vi "disable all controls.vi"(6 "DisabledEnum":T1(ring)=enum."Disabled and Grayed Out", 8 "error in":errorcluster, 11 "Cluster in":T2={"This VI Ref"=refnum, "Test VI"=refnum, "Q Ref"=refnum, "UE"=refnum, "Data"=variant, "Timeout"=-1, "Path List[]"=[], "Status"="", "Counter"=0, "Config"={"Source Path"=path "", "Dest Path"=path "", "Log Path"=path "", "Move?"=FALSE, "Log?"=FALSE, "Scanners"=[], "Excude Folders"=[], "Jpg?"=FALSE, "Default path"=path "", "Extended?"=FALSE, "Mode"=enum."Move", "Temp"=FALSE}, "Total"=0, "Config Path"=path "", "exif info"={"Make"="Canon\u0000", "Model"="Canon PowerShot A495\u0000", "Orientation"=0, "Date"=timestamp(0 s since 1904-01-01), "Width"=0, "Height"=0, "Square?"=FALSE, "File Name"="Canon\u0000", "Extension"="Canon\u0000", "Valid?"=FALSE, "Path"=path "", "size"=0, "No Ext?"=FALSE, "prefix?"=FALSE, "String"="", "Name Type"=enum."Event Sufix"}, "app operation"=enum."Start", "Log Ref"=refnum, "Start Time"=0.0, "Pause Time"=0.0, "Argument?"=FALSE, "Argument path"=path "", "Identical"=FALSE, "File.lvclass"=refnum}) -> (0 "error out":errorcluster, 3 "Cluster out":T2={"This VI Ref"=refnum, "Test VI"=refnum, "Q Ref"=refnum, "UE"=refnum, "Data"=variant, "Timeout"=-1, "Path List[]"=[], "Status"="", "Counter"=0, "Config"={"Source Path"=path "", "Dest Path"=path "", "Log Path"=path "", "Move?"=FALSE, "Log?"=FALSE, "Scanners"=[], "Excude Folders"=[], "Jpg?"=FALSE, "Default path"=path "", "Extended?"=FALSE, "Mode"=enum."Move", "Temp"=FALSE}, "Total"=0, "Config Path"=path "", "exif info"={"Make"="Canon\u0000", "Model"="Canon PowerShot A495\u0000", "Orientation"=0, "Date"=timestamp(0 s since 1904-01-01), "Width"=0, "Height"=0, "Square?"=FALSE, "File Name"="Canon\u0000", "Extension"="Canon\u0000", "Valid?"=FALSE, "Path"=path "", "size"=0, "No Ext?"=FALSE, "prefix?"=FALSE, "String"="", "Name Type"=enum."Event Sufix"}, "app operation"=enum."Start", "Log Ref"=refnum, "Start Time"=0.0, "Pause Time"=0.0, "Argument?"=FALSE, "Argument path"=path "", "Identical"=FALSE, "File.lvclass"=refnum})   [LabVIEW 2023, in "User Interface.lvlib"]
uses:
  User Interface.lvlib
  Controls/configuration cluster.ctl
  File Classes/Controls/rename type enum.ctl
  File Classes/File Classes.lvlib
  File Classes/Controls/exif data cluster.ctl
  Controls/app operation state enum.ctl
  File Classes/File/File.lvclass
  Controls/main consumer cluster.ctl
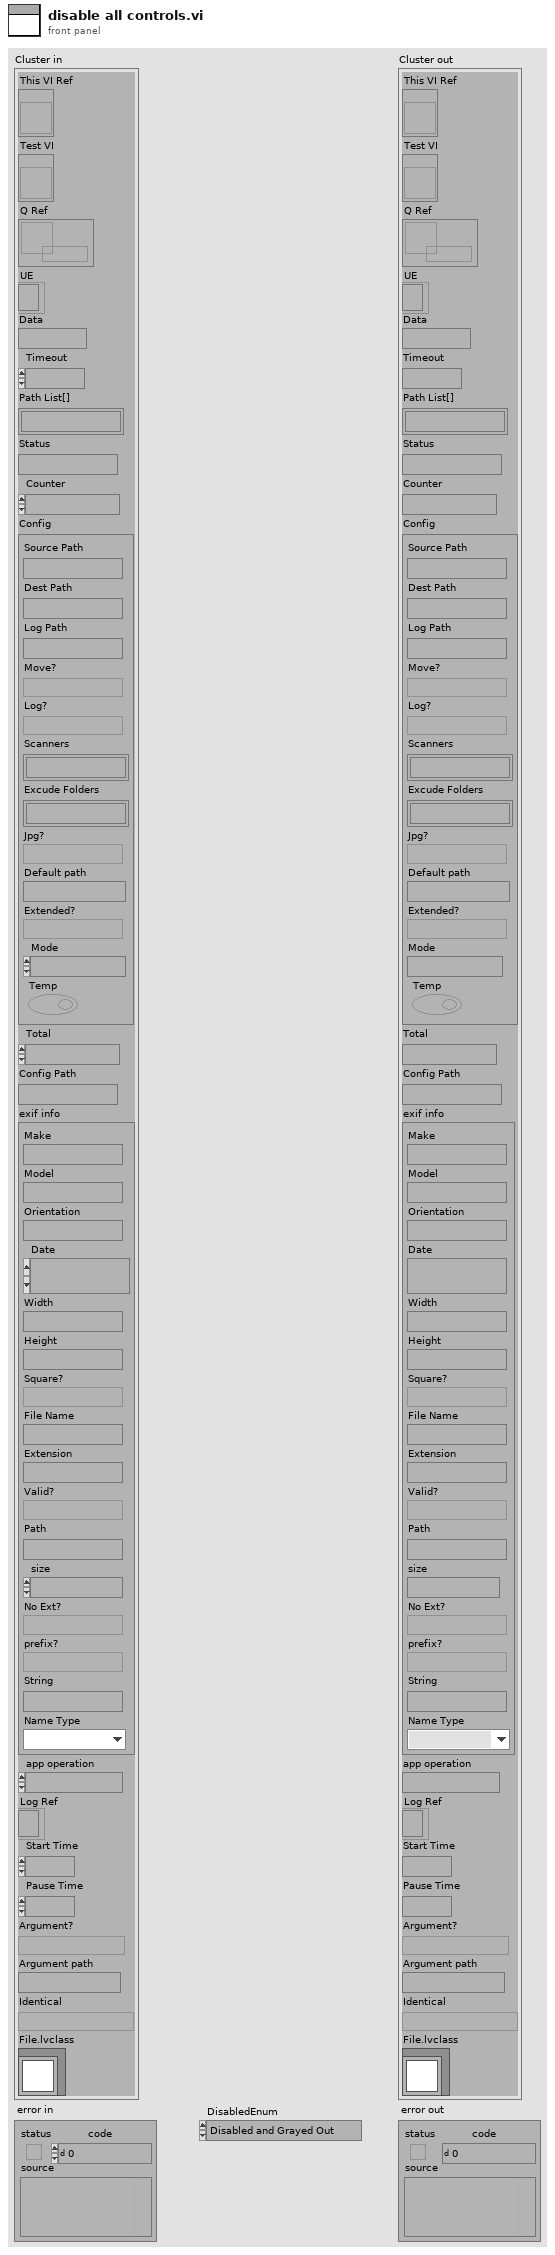
[diagram p1: front panel]
types:
  T1 = enum8{"Enabled", "Disabled", "Disabled and Grayed Out"}
  T2 = typedef "User Interface.lvlib/main consumer cluster.ctl" = cluster{"This VI Ref":refnum<vi>, "Test VI":refnum<vi>, "Q Ref":refnum<queue>, "UE":refnum<event-registration>, "Data":variant, "Timeout":i32, "Path List[]":path[], "Status":string, "Counter":i32, "Config":T3, "Total":i32, "Config Path":path, "exif info":T4, "app operation":T6, "Log Ref":refnum<file>, "Start Time":dbl, "Pause Time":dbl, "Argument?":bool, "Argument path":path, "Identical":bool, "File.lvclass":refnum<class "File.lvclass">}
  T3 = typedef "User Interface.lvlib/configuration cluster.ctl" = cluster{"Source Path":path, "Dest Path":path, "Log Path":path, "Move?":bool, "Log?":bool, "Scanners":string[], "Excude Folders":string[], "Jpg?":bool, "Default path":path, "Extended?":bool, "Mode":enum16{"Copy (Default)", "Move", "Rename"}, "Temp":bool}
  T4 = typedef "File Classes.lvlib/exif data cluster.ctl" = cluster{"Make":string, "Model":string, "Orientation":u16, "Date":timestamp, "Width":u16, "Height":u16, "Square?":bool, "File Name":string, "Extension":string, "Valid?":bool, "Path":path, "size":i64, "No Ext?":bool, "prefix?":bool, "String":string, "Name Type":T5}
  T5 = typedef "File Classes.lvlib/rename type enum.ctl" = enum16{"Date & Time (Default)", "Model Sufix", "Event Sufix", "Model & Event Sufix"}
  T6 = typedef "User Interface.lvlib/app operation state enum.ctl" = enum16{"Start", "Stop", "Pause", "Resume"}
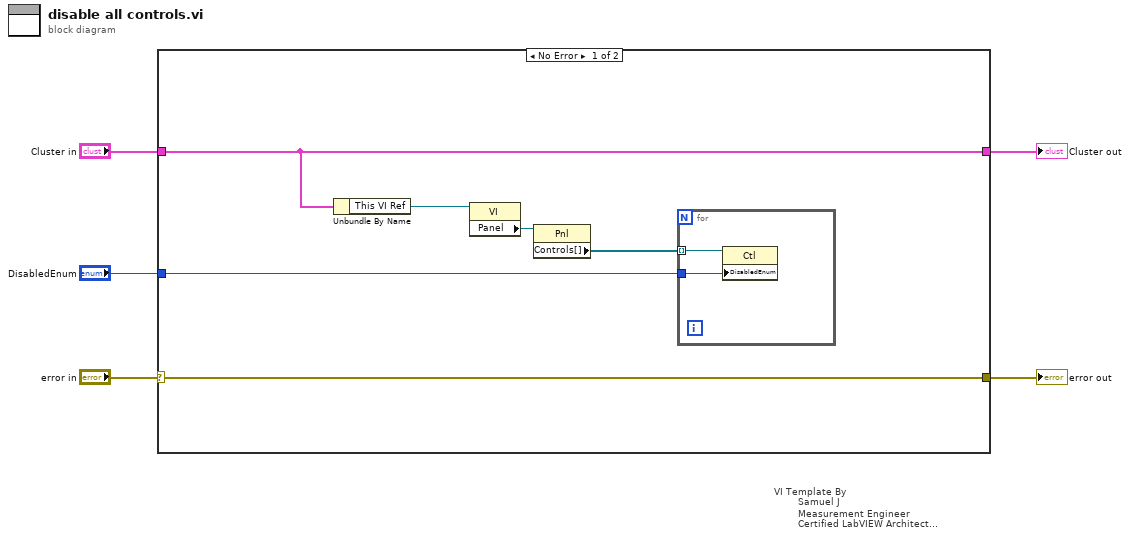
[diagram p0: block diagram]
diagram:
  n1 = case "VI Template By\n        Samuel J\n        Measurement Engineer\n        Certified LabVIEW Architect\n        Vestas Technology R&D Chennai" shown="No Error" "error in" {
    selector: "error in" -> [w11 w15]
    tunnel: [w11 w15] -> w4
    tunnel: "Cluster in" -> [w9 w14]
    tunnel: [w9 w14] -> w2
    tunnel: "DisabledEnum" -> [w6 _]
    frame No Error {
      n2 = Unbundle By Name(w9) -> ("This VI Ref"=w7:refnum<vi>)
      n3 = property class="VI"(reference=w7) -> ("Panel"=w10:refnum<vi>)  [unwired: 1 in, 2 out]
      n4 = property class="Pnl"(reference=w10) -> ("Controls[]"=w8:refnum<vi>[])  [unwired: 1 in, 2 out]
      n5 = for {
        tunnel: w8 -> [w13] mode=indexing
        tunnel: w6 -> [w12]
        n6 = property class="Ctl"(reference=w13, "DisabledEnum"=w12) -> ()  [unwired: 1 in, 2 out]
      }
    }
    frame Error {
    }
  }
  "error out" <- w4
  "Cluster out" <- w2
